vi "Get_link_info.vi"(0 "VI Name":string) -> (1 "Server IP & Port":string, 2 "Path name":path, 3 "Application reference":refnum<vi>, 4 "Local Call?":bool)   [LabVIEW 2010]
uses:
  Anemometry/Anemometry Sub Vis/Controls/Serveds.ctl
  Anemometry/Anemometry Sub Vis/Controls/App_Global.ctl
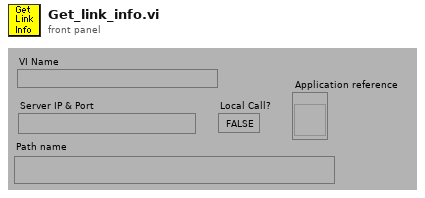
[diagram p1: front panel]
types:
  T1 = typedef "Serveds.ctl" = enum16{"Read Global", "Load Global From File"}
  T2 = typedef "App_Global.ctl" = enum16{"Read Global", "Write to Global", "Initialise Array"}
  T3 = typedef "App_Ref_Cluster.ctl" = cluster{"Server IP & Port No":string, "Application reference":refnum<vi>}
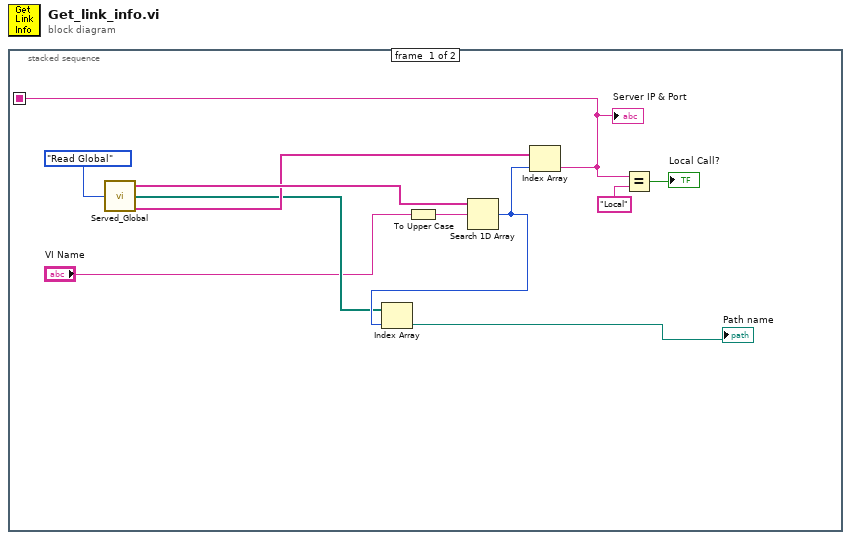
[diagram p0: block diagram]
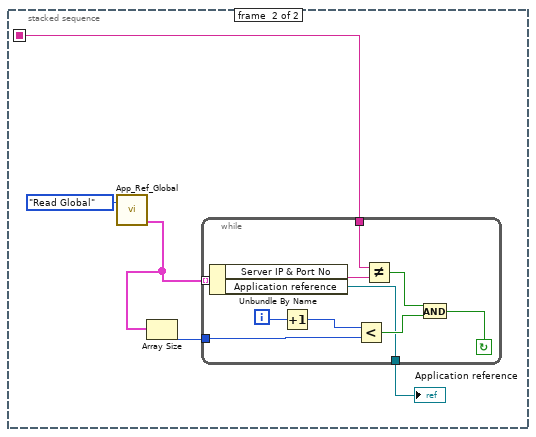
[diagram p2: hidden frame]
diagram:
  n1 = stacked-sequence {
    seq-local: [w8 _] -> [_ w12]
    frame #0 {
      n2 = call "Served_Global.vi"("Mode"=Serveds."Read Global") -> ("Served VI Name"=w7:string[], "Served VI Path"=w5:path[], "Served IP Number & Port No"=w6:string[])
      n3 = To Upper Case(1:"VI Name") -> (0:w1:string)
      n4 = Search 1D Array(1D array=w7, element=w1) -> (index of element=w11:i32)  [unwired: 1 out]
      n5 = Index Array(array=w5, index=w11) -> (element=→"Path name":path)
      n6 = Index Array(array=w6, index=w11) -> (element=w8:string)
      "Server IP & Port" <- w8
      n7 = Equal?(x=w8, y="Local" ("t")) -> (x = y?=→"Local Call?":bool)
    }
    frame #1 {
      n8 = call "App_Ref_Global.vi"("Mode"=App_Global."Read Global") -> ("Output Array"=w15:T3[])  [unwired: 1 in, 1 out]
      n9 = Array Size(array=w15) -> (size(s)=w14:i32)
      n10 = while {
        tunnel: [w17] -> w13
        tunnel: w14 -> [w22]
        tunnel: w12 -> [w24]
        tunnel: w15 -> [w26] mode=indexing
        i -> [w23]
        stop <- w18 continue-if-true
        n11 = Unbundle By Name(w26) -> ("Server IP & Port No"=w25:string, "Application reference"=w17:refnum<vi>)
        n12 = Increment(x=w23) -> (x+1=w21:i32)
        n13 = Less?(x=w21, y=w22) -> (x < y?=w20:bool)
        n14 = Not Equal?(x=w24, y=w25) -> (x != y?=w19:bool)
        n15 = And(x=w19, y=w20) -> (x .and. y?=w18:bool)
      }
      "Application reference" <- w13
    }
  }
